vi "przypisz skale Y.vi"(7 "modyf skali (2)":i32=2, 8 "error in (no error)":errorcluster, 9 "szukany zakres in":dbl, 10 "Zakresy we":cluster{"Zakresy":dbl[], "skale":i32[]}) -> (0 "error out":errorcluster, 2 "Zakresy wy":cluster{"Zakresy":dbl[], "skale":i32[]}, 3 "skala wy":i32)   [LabVIEW 2014]
doc: "Przypisuje skale Y na podstawie zakresu pomiarowego\n(wykrywa czy podany zakres zosta³ wczeœniej przypisany do skali)"
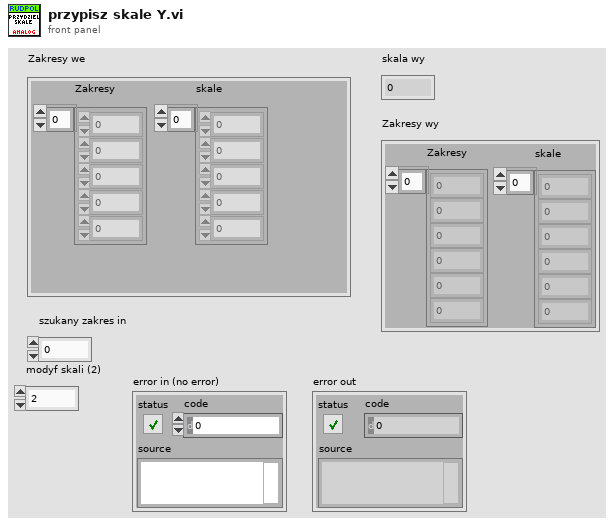
[diagram p1: front panel]
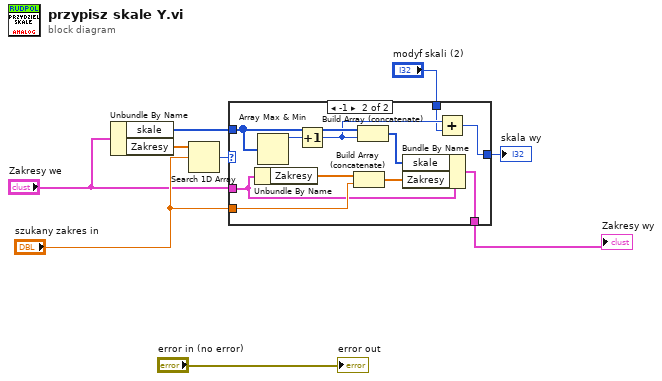
[diagram p0: block diagram]
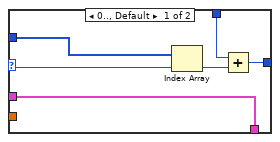
[diagram p2: hidden frame]
diagram:
  n1 = Unbundle By Name("Zakresy we") -> ("skale"=w4:i32[], "Zakresy"=w8:dbl[])
  n2 = Search 1D Array(1D array=w8, element="szukany zakres in") -> (index of element=w9:i32)  [unwired: 1 in]
  n3 = case shown="-1" w9 {
    selector: w9 -> [w15 _]
    tunnel: w4 -> [w14 w25]
    tunnel: [w12 w18] -> w6
    tunnel: "Zakresy we" -> [w13 w20]
    tunnel: "szukany zakres in" -> [_ w22]
    tunnel: [w13 w17] -> w5
    tunnel: "modyf skali (2)" -> [w10 w16]
    frame 0.., Default {
      n4 = Index Array(array=w14, index=w15) -> (element=w11:i32)
      n5 = Add(x=w10, y=w11) -> (x+y=w12:i32)
    }
    frame -1 {
      n6 = Unbundle By Name(w20) -> ("Zakresy"=w23:dbl[])
      n7 = Array Max & Min(array=w25) -> (max value=w26:i32)  [unwired: 3 out]
      n8 = Increment(x=w26) -> (x+1=w19:i32)
      n9 = Build Array (concatenate)(w23, w22) -> (w21:dbl[])
      n10 = Build Array (concatenate)(w25, w19) -> (w24:i32[])
      n11 = Bundle By Name(cluster=w20, "skale"=w24, "Zakresy"=w21) -> (w17:cluster{"Zakresy":dbl[], "skale":i32[]})
      n12 = Add(x=w19, y=w16) -> (x+y=w18:i32)
    }
  }
  "Zakresy wy" <- w5
  "skala wy" <- w6
  "error out" <- "error in (no error)"
